vi "Module Cleanup.vi"(8 "error in (no error)":errorcluster, 11 "Config Updater Module in":refnum<class "Git Updater Module.lvclass">) -> (0 "error out":errorcluster, 3 "Config Updater Module out":refnum<class "Git Updater Module.lvclass">)   [LabVIEW 2020, in "Volatus.lvlib" / "Git Updater Module.lvclass"]
uses:
  Git Updater Module.lvclass
  Git Updater Module.lvclass/Git Updater Module.ctl
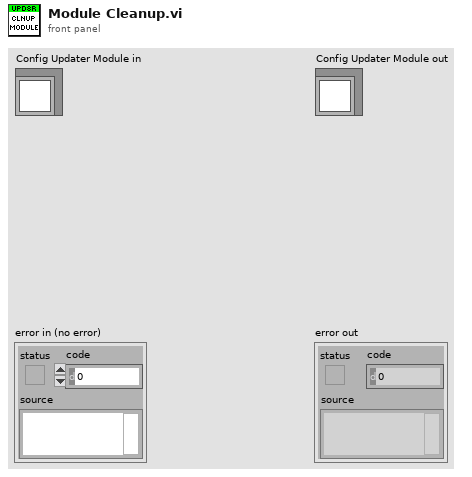
[diagram p1: front panel]
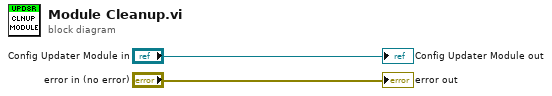
[diagram p0: block diagram]
diagram:
  "error out" <- "error in (no error)"
  "Config Updater Module out" <- "Config Updater Module in"
